vi "Data entry form multi-module.vi"(8 "error in (no error)":errorcluster, 9 "Assembly Type":string, 10 "Is Module?":bool, 11 "Database Entry in":refnum<class "Database Entry.lvclass">) -> (0 "error out":errorcluster, 1 "Is Dummy run?":bool, 2 "Aborted":bool, 3 "Database Entry out":refnum<class "Database Entry.lvclass">)   [LabVIEW 2021, in "Database Entry.lvclass"]
uses:
  Database Entry.lvclass
  Database Entry.lvclass/Database Entry.ctl
  Components/Stack/Stack.lvclass
panel:
  out "RingText.Text":string
  out "Now assembling...":string
  in  "Protomodule Steps":T1(ring)
  in  "Module Steps":T2(ring)
  in  "Dummy run submit":bool
  out "Use same values for both":bool
  in  "Use same values for all":bool
  out "Instructions":string
  in  "Module Instuctions":T3(ring)
  in  "Protomodule Instructions":T4(ring)
  in  "Submit":bool
  in  "Gantry":T5
  out "Stage":string
  in  "Steps":T6(ring)
  in  "Abort":bool
  in  "Next":bool
  in  "Previous":bool
  # "Col 1"
  # "Col 2"
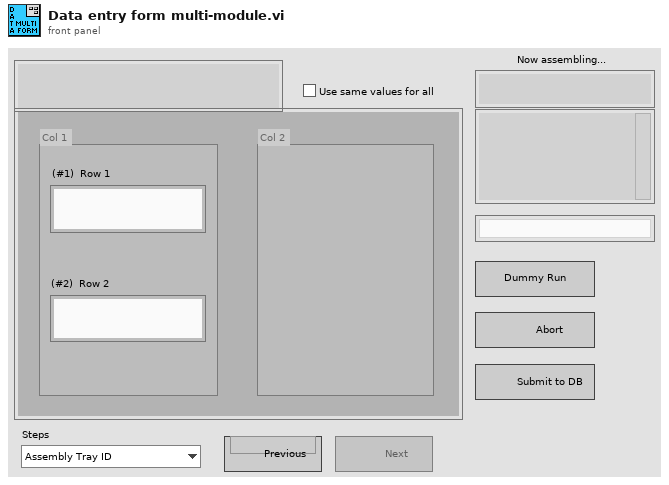
[diagram p1: front panel]
types:
  T1 = enum16{"Assembly Tray ID", "Module Stack ID", "Baseplate ID", "Sensor PUT ID", "Sensor Tray ID", "Sensor ID", "Sensor grade", "Comments", "Glue batch number", "Tape batch number"}
  T2 = enum16{"Assembly Tray ID", "Module Stack ID", "Protomodule ID", "Hexaboard PUT ID", "Hexaboard Tray ID", "Hexaboard ID", "Sensor grade", "Comments", "Glue batch number", "Tape batch number"}
  T3 = enum16{"Assembly Tray ID is always required.                For dummy runs, skip entry of other data.", "Scan the MODULE QR code (320M).                 **Leave blank for dummy runs**", "Verify the protomodule ID (320P) or scan the module QR code.                 **Leave blank for dummy runs**", "Hexaboard pick-up-tool ID", "Hexaboard Tray ID", "Scan the hexaboard QR code (320XL).                 **Leave blank for dummy runs**", "(Optional) Leave blank if no updated grade for the sensor", "Comments, if any.", "Glue batch number", "Tape batch number"}
  T4 = enum16{"Assembly Tray ID is always required.                For dummy runs, skip entry of other data.", "Scan the MODULE QR code (320M) for this protomodule.                 **Leave blank for dummy runs**", "Scan the baseplate QR code (320BA).                 **Leave blank for dummy runs**", "Sensor pick-up-tool ID", "Sensor Tray ID", "Scan the sensor barcode.                 **Leave blank for dummy runs**", "Sensor grade (default A)", "Include sensor visual inspection comments here.", "Glue batch number", "(Optional) Tape batch number"}
  T5 = cluster{"(#1)  Row 1":string, "(#2)  Row 2":string, "(#3)  Row 1":string, "(#4)  Row 2":string}
  T6 = enum16{"Assembly Tray ID", "Module Stack ID", "Base-layer (BP/PL) ID", "Pick-up-tool ID", "Component Tray ID", "Top-layer (Sen/Hxb) ID", "Sensor grade", "Comments", "Glue batch number"}
  T7 = enum8{"Enabled", "Disabled", "Disabled and Grayed Out"}
  T8 = enum16{"Assembly Tray ID", "Module Stack ID", "Base-layer (BP/PL) ID", "Pick-up-tool ID", "Component Tray ID", "Top-layer (Sen/Hxb) ID", "Sensor grade", "Comments", "Glue batch number", "Tape batch number"}
  T9 = cluster{"(#1)  Pos 1":string, "(#2)  Pos 2":string, "(#3)  Pos 1":string, "(#4)  Pos 2":string}
  T10 = cluster{"Value[0]":string, "Value[1]":string, "Value[2]":string, "Value[3]":string}
  T11 = cluster{"[0]":string, "[1]":string, "[2]":string, "[3]":string}
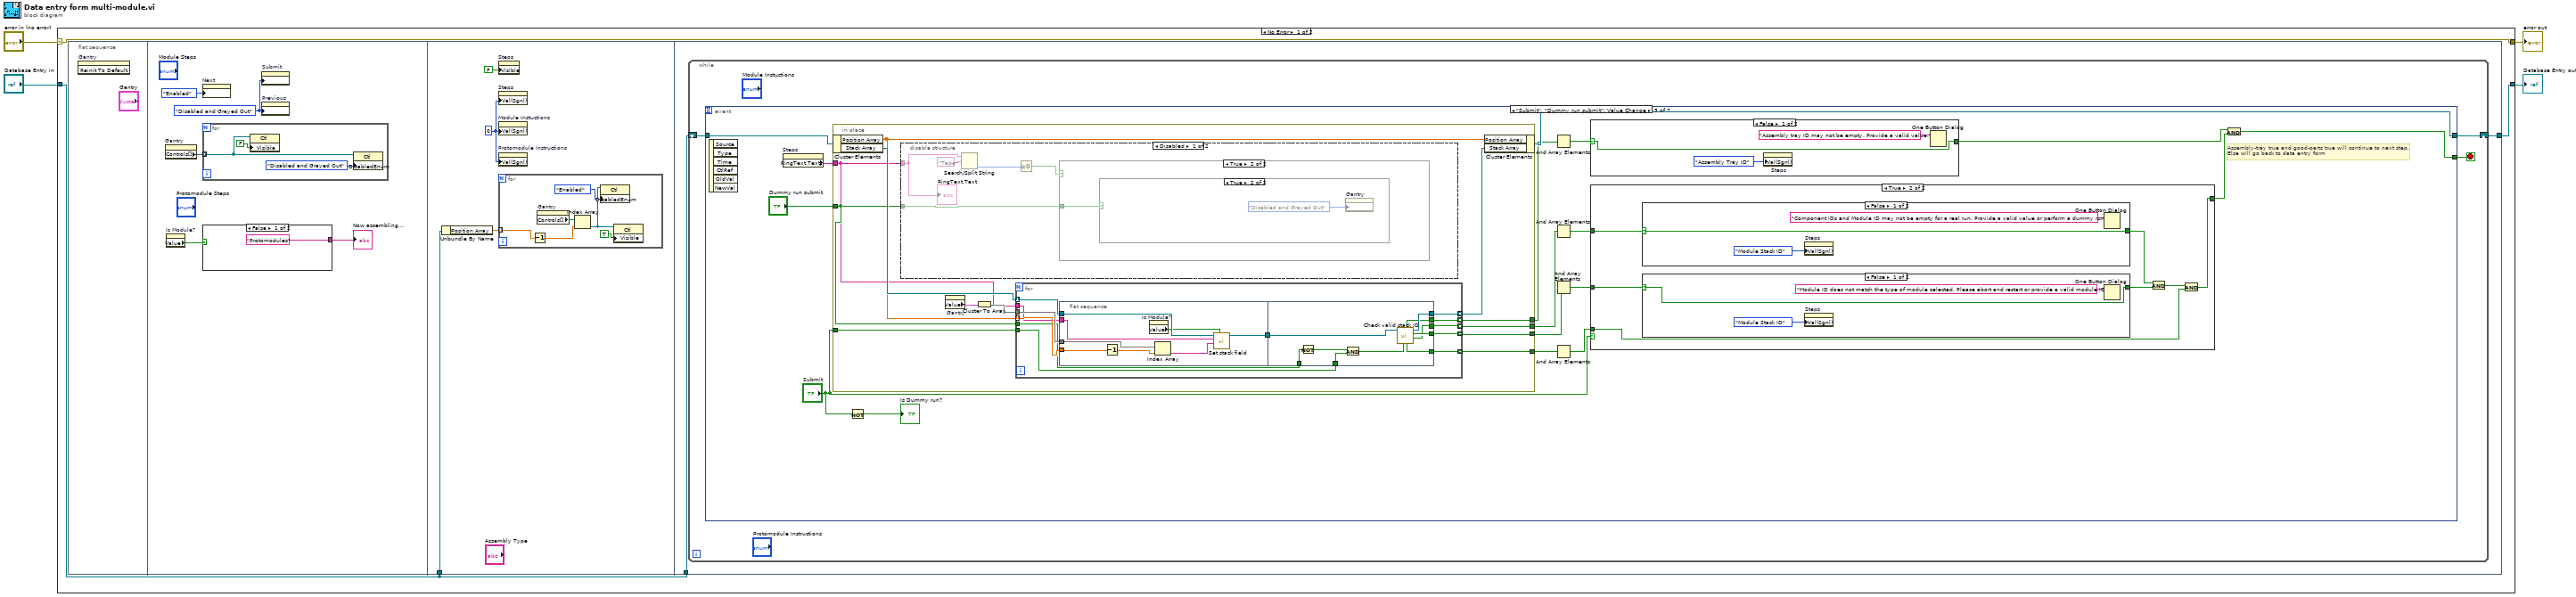
[diagram p0: block diagram]
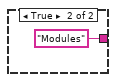
[diagram p2: hidden frame]
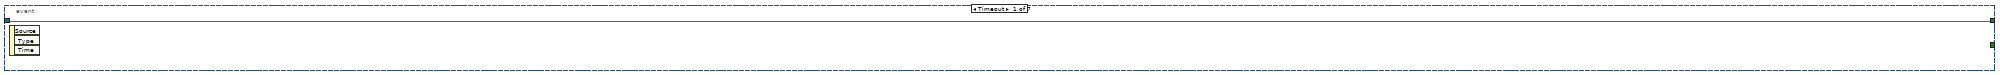
[diagram p3: hidden frame]
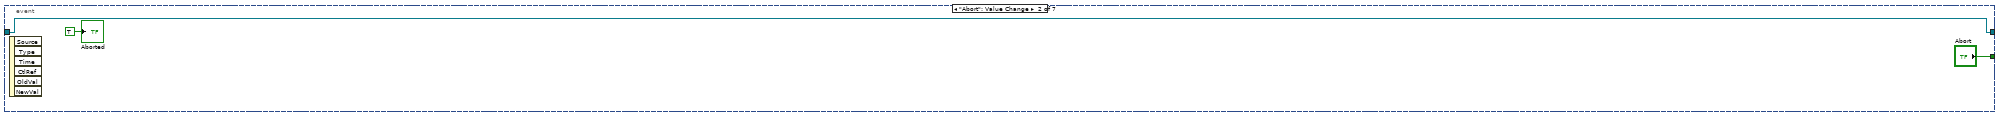
[diagram p4: hidden frame]
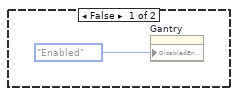
[diagram p5: hidden frame]
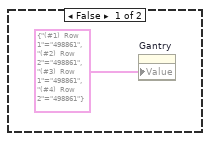
[diagram p6: hidden frame]
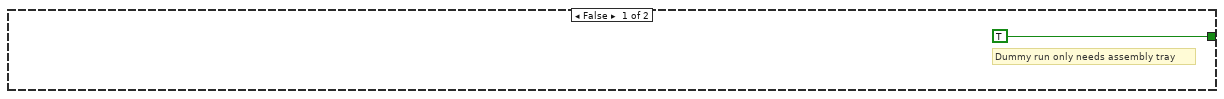
[diagram p8: hidden frame]
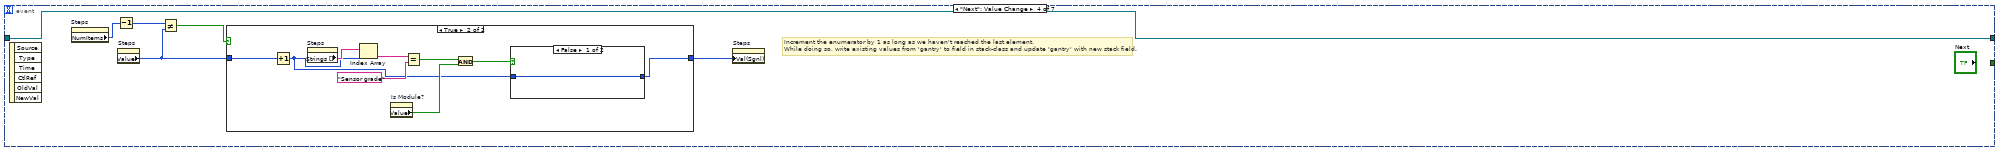
[diagram p12: hidden frame]
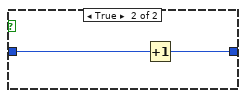
[diagram p14: hidden frame]
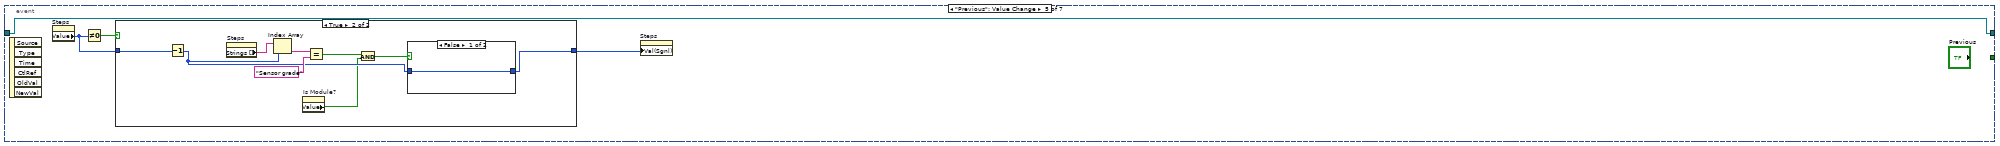
[diagram p15: hidden frame]
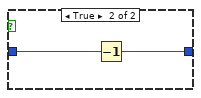
[diagram p17: hidden frame]
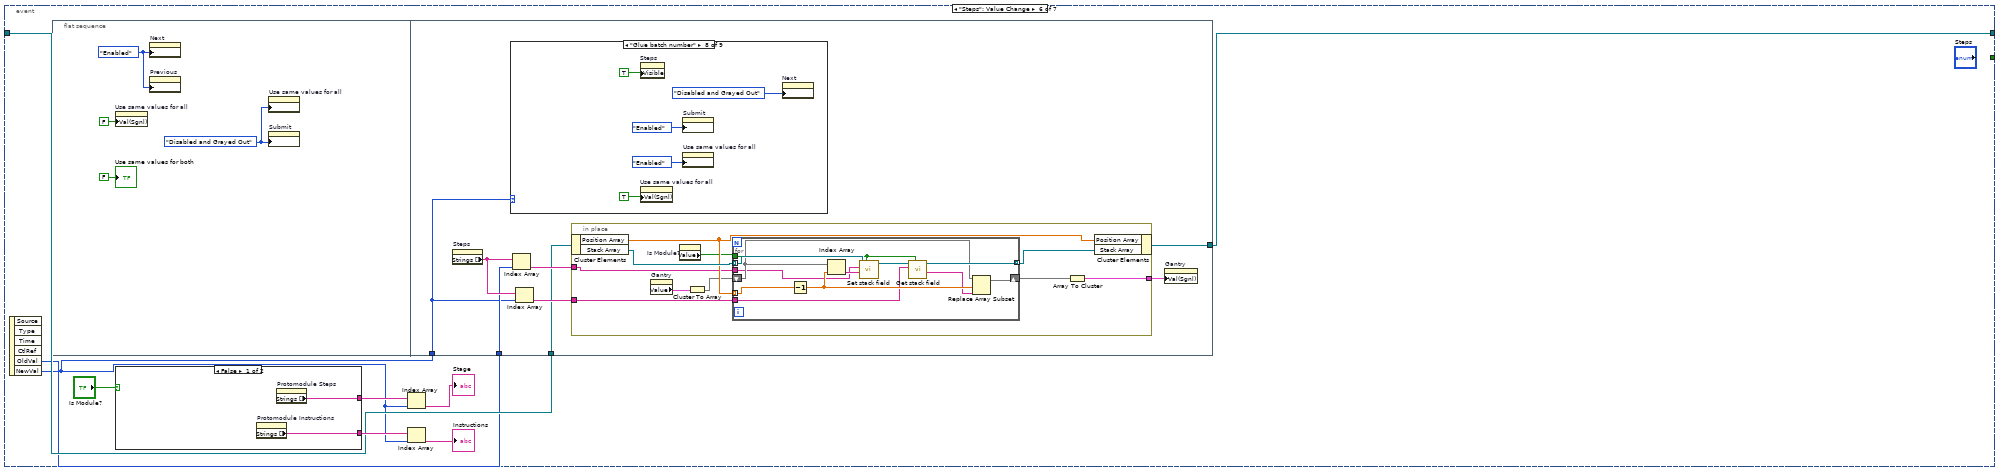
[diagram p18: hidden frame]
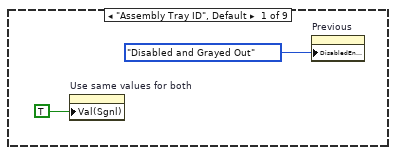
[diagram p19: hidden frame]
diagram:
  n1 = case shown="No Error" "error in (no error)" {
    selector: "error in (no error)" -> [w7 w298]
    tunnel: [w7 w298] -> w3
    tunnel: "Database Entry in" -> [w5 w297]
    tunnel: [w6 w297] -> w1
    frame No Error {
      n2 = flat-sequence {
        tunnel: w5 -> [w19]
        tunnel: w5 -> [w28]
        tunnel: [w29] -> w6
        frame #0 {
          n3 = invoke on="Gantry" class="Clust (strict)" method="Reinit To Default"() -> ()  [unwired: 3 in, 3 out]
        }
        frame #1 {
          w11 = T7."Disabled and Grayed Out" ("Disabled")
          n4 = property on="Gantry" class="Clust (strict)"() -> ("Controls[]"=w12:refnum<vi>[])  [unwired: 2 in, 2 out]
          n5 = property on="Is Module?" class="Bool (strict)"() -> ("Value"=w8:bool)  [unwired: 2 in, 2 out]
          n6 = property on="Next" class="Bool"("DisabledEnum"=T7."Enabled" ("Disabled")) -> ()  [unwired: 2 in, 2 out]
          n7 = for {
            tunnel: w12 -> [w15] mode=indexing
            n8 = property class="Ctl"(reference=w15, "Visible"=FALSE) -> ()  [unwired: 1 in, 2 out]
            n9 = property class="Ctl"(reference=w15, "DisabledEnum"=T7."Disabled and Grayed Out" ("Disabled")) -> ()  [unwired: 1 in, 2 out]
          }
          n10 = case shown="False" w8 {
            tunnel: ["Protomodules" ("Now assembling...") "Modules" ("Now assembling...")] -> w9
            frame False {
            }
            frame True {
            }
          }
          "Now assembling..." <- w9
          n11 = property on="Submit" class="Bool"("DisabledEnum"=w11) -> ()  [unwired: 2 in, 2 out]
          n12 = property on="Previous" class="Bool"("DisabledEnum"=w11) -> ()  [unwired: 2 in, 2 out]
        }
        frame #2 {
          w20 = u16 0 ("Value (Signaling)")
          n13 = Unbundle By Name(w19) -> ("Position Array"=w18:dbl[])
          n14 = property on="Steps" class="Enum (strict)"("Visible"=FALSE) -> ()  [unwired: 2 in, 2 out]
          n15 = property on="Steps" class="Enum (strict)"("Val(Sgnl)"=w20) -> ()  [unwired: 2 in, 2 out]
          n16 = property on="Module Instuctions" class="Enum (strict)"("Val(Sgnl)"=w20) -> ()  [unwired: 2 in, 2 out]
          n17 = property on="Protomodule Instructions" class="Enum (strict)"("Val(Sgnl)"=w20) -> ()  [unwired: 2 in, 2 out]
          n18 = for {
            tunnel: w18 -> [w23] mode=indexing
            n19 = Decrement(x=w23) -> (x-1=w22:dbl)
            n20 = property on="Gantry" class="Clust (strict)"() -> ("Controls[]"=w27:refnum<vi>[])  [unwired: 2 in, 2 out]
            n21 = Index Array(array=w27, index=w22) -> (element=w25:refnum<vi>)
            n22 = property class="Ctl"(reference=w25, "DisabledEnum"=T7."Enabled" ("Disabled")) -> ()  [unwired: 1 in, 2 out]
            n23 = property class="Ctl"(reference=w25, "Visible"=TRUE) -> ()  [unwired: 1 in, 2 out]
          }
        }
        frame #3 {
          n24 = while {
            shift-right: [w31] -> w29
            shift-left: w28 -> [w30]
            stop <- w32 stop-if-true
            # "While loop"
            n25 = event shown="[2] \"Submit\", \"Dummy run submit\": Value Change" {
              selector: _ -> [_ _ _ _ _ _ _]
              dyn-events: _ -> [_ _ _ _ _ _ _]
              timeout: _ -> [_ _ _ _ _ _ _]
              tunnel: [_ "Abort" w42 _ _ _ _] -> w32
              tunnel: w30 -> [w33 w35 w53 w125 w144 w164 w216]
              tunnel: [w33 w35 w52 w125 w144 w163 w216] -> w31
              event Timeout {
                n26 = event-data() -> ()  [unwired: 1 in, 3 out]
              }
              event "Abort": Value Change {
                n27 = event-data() -> ()  [unwired: 1 in, 6 out]
                "Aborted" <- TRUE ("Aborted")
              }
              event "Submit", "Dummy run submit": Value Change {
                # "Assembly-tray true and good-parts true will continue to next step. \nElse will go back to data entry form"
                n28 = event-data() -> ()  [unwired: 1 in, 6 out]
                n29 = property on="Steps" class="Enum (strict)"() -> ("RingText.Text"=w48:string)  [unwired: 2 in, 2 out]
                n30 = in-place {
                  in-place-border: w48 -> [w54]
                  in-place-border: [w60] -> w51
                  in-place-border: [w59] -> w50
                  in-place-border: [w58] -> w49
                  in-place-border: "Dummy run submit" -> [w57]
                  in-place-border: "Submit" -> [w56]
                  in-place-border: [w55] -> w38
                  n31 = in-place-cluster #1(w53) -> ("Position Array"=w64:dbl[], "Stack Array"=w65:refnum<class "Stack.lvclass">[])
                  n32 = disable-structure shown="Disabled" {
                    disable-tunnel: w57 -> [w70 _]
                    disable-tunnel: w54 -> [w69 _]
                    frame Disabled {
                      n33 = Search/Split String(string=w69, search string/char (-)="Tape") -> (offset of match=w67:i32)  [unwired: 1 in, 2 out]
                      n34 = Greater Or Equal To 0?(x=w67) -> (x >= 0?=w66:bool)
                      n35 = case shown="True" w66 {
                        tunnel: w70 -> [_ w72]
                        frame False {
                          n36 = property on="Gantry" class="Clust (strict)"("DisabledEnum"=T7."Enabled" ("Disabled")) -> ()  [unwired: 2 in, 2 out]
                        }
                        frame True {
                          n37 = case shown="True" w72 {
                            frame False {
                              n38 = property on="Gantry" class="Clust (strict)"("Value"=T5 {"(#1)  Row 1"="498861", "(#2)  Row 2"="498861", "(#3)  Row 1"="498861", "(#4)  Row 2"="498861"} ("Gantry")) -> ()  [unwired: 2 in, 2 out]
                            }
                            frame True {
                              n39 = property on="Gantry" class="Clust (strict)"("DisabledEnum"=T7."Disabled and Grayed Out" ("Disabled")) -> ()  [unwired: 2 in, 2 out]
                            }
                          }
                        }
                      }
                      "RingText.Text" <- w69
                    }
                    frame Enabled {
                    }
                  }
                  n40 = property on="Gantry" class="Clust (strict)"() -> ("Value"=w62:T9)  [unwired: 2 in, 2 out]
                  n41 = Cluster To Array(cluster=w62) -> (array=w63:string[])
                  n42 = for {
                    tunnel: w65 -> [w86] mode=indexing
                    tunnel: w64 -> [w85] mode=indexing
                    tunnel: [w83] -> w61 mode=indexing
                    tunnel: w54 -> [w76]
                    tunnel: w63 -> [w84]
                    tunnel: w56 -> [w81]
                    tunnel: w57 -> [w75]
                    tunnel: [w80] -> w60 mode=indexing
                    tunnel: [w79] -> w59 mode=indexing
                    tunnel: [w78] -> w58 mode=indexing
                    tunnel: [w77] -> w55 mode=indexing
                    n43 = flat-sequence {
                      tunnel: w86 -> [w94]
                      tunnel: w85 -> [w93]
                      tunnel: w84 -> [w91]
                      tunnel: w76 -> [w89]
                      tunnel: [w88] -> w82
                      tunnel: [w103] -> w83
                      tunnel: w82 -> [w104]
                      tunnel: w81 -> [w101]
                      tunnel: w75 -> [w100]
                      tunnel: [w98] -> w80
                      tunnel: [w97] -> w79
                      tunnel: [w96] -> w78
                      tunnel: [w95] -> w77
                      frame #0 {
                        n44 = Decrement(x=w93) -> (x-1=w90:dbl)
                        n45 = property on="Is Module?" class="Bool (strict)"() -> ("Value"=w87:bool)  [unwired: 2 in, 2 out]
                        n46 = Index Array(array=w91, index=w90) -> (element=w92:string)
                        n47 = call "Set stack field.vi"("Is Module?"=w87, "Value in"=w92, "Field"=w89, "Stack in"=w94) -> ("Stack out"=w88:refnum<class "Stack.lvclass">)  [unwired: 6 in, 1 out]
                      }
                      frame #1 {
                        n48 = Not(x=w100) -> (.not. x?=w99:bool)
                        n49 = And(x=w99, y=w101) -> (x .and. y?=w102:bool)
                        n50 = call "Check valid stack ID.vi"("Is real run?"=w102, "Stack in"=w104) -> ("Non-empty part IDs?"=w97:bool, "Valid module ID?"=w98:bool, "Stack out"=w103:refnum<class "Stack.lvclass">, "Continue with current parts"=w95:bool, "Non-empty assembly tray ID?"=w96:bool)  [unwired: 4 in, 1 out]
                      }
                    }
                  }
                  n51 = in-place-cluster #1("Position Array"=w64, "Stack Array"=w61) -> (w52:refnum<class "Database Entry.lvclass">)
                }
                n52 = Not(x="Submit") -> (.not. x?=→"Is Dummy run?":bool)
                n53 = And Array Elements(Boolean array=w49) -> (logical AND=w47:bool)
                n54 = And Array Elements(Boolean array=w50) -> (logical AND=w46:bool)
                n55 = And Array Elements(Boolean array=w51) -> (logical AND=w44:bool)
                n56 = And Array Elements(Boolean array=w38) -> (logical AND=w37:bool)
                n57 = case shown="False" w47 {
                  selector: w47 -> [w122 w124]
                  tunnel: [w122 w124] -> w43
                  frame False {
                    n58 = property on="Steps" class="Enum (strict)"("Val(Sgnl)"=T8."Assembly Tray ID" ("Value (Signaling)")) -> ()  [unwired: 2 in, 2 out]
                    n59 = One Button Dialog(message="Assembly tray ID may not be empty. Provide a valid value.") -> ()  [unwired: 1 in, 1 out]
                  }
                  frame True {
                  }
                }
                n60 = case shown="True" "Submit" {
                  tunnel: w46 -> [_ w112]
                  tunnel: w44 -> [_ w111]
                  tunnel: [TRUE w106] -> w41
                  tunnel: w37 -> [_ w108]
                  frame False {
                    # "Dummy run only needs assembly tray"
                  }
                  frame True {
                    n61 = case shown="False" w112 {
                      selector: w112 -> [w118 w120]
                      tunnel: [w118 w120] -> w110
                      frame False {
                        n62 = property on="Steps" class="Enum (strict)"("Val(Sgnl)"=T8."Module Stack ID" ("Value (Signaling)")) -> ()  [unwired: 2 in, 2 out]
                        n63 = One Button Dialog(message="Component IDs and Module ID may not be empty for a real run. Provide a valid value or perform a dummy run.") -> ()  [unwired: 1 in, 1 out]
                      }
                      frame True {
                      }
                    }
                    n64 = case shown="False" w111 {
                      selector: w111 -> [w114 w116]
                      tunnel: [w114 w116] -> w109
                      frame False {
                        n65 = property on="Steps" class="Enum (strict)"("Val(Sgnl)"=T8."Module Stack ID" ("Value (Signaling)")) -> ()  [unwired: 2 in, 2 out]
                        n66 = One Button Dialog(message="Module ID does not match the type of module selected. Please abort and restart or provide a valid module ID.") -> ()  [unwired: 1 in, 1 out]
                      }
                      frame True {
                      }
                    }
                    n67 = And(x=w110, y=w109) -> (x .and. y?=w107:bool)
                    n68 = And(x=w107, y=w108) -> (x .and. y?=w106:bool)
                  }
                }
                n69 = And(x=w43, y=w41) -> (x .and. y?=w42:bool)
              }
              event "Next": Value Change {
                # "Increment the enumerator by 1 as long as we haven't reached the last element.\nWhile doing so, write existing values from 'gantry' to field in stack-class and update 'gantry' with new stack field."
                n70 = event-data() -> ()  [unwired: 1 in, 6 out]
                n71 = property on="Steps" class="Enum (strict)"() -> ("NumItems"=w130:u32)  [unwired: 2 in, 2 out]
                n72 = Decrement(x=w130) -> (x-1=w129:u32)
                n73 = property on="Steps" class="Enum (strict)"() -> ("Value"=w127:T6)  [unwired: 2 in, 2 out]
                n74 = Not Equal?(x=w129, y=w127) -> (x != y?=w128:bool)
                n75 = case shown="True" w128 {
                  tunnel: w127 -> [w131 w140]
                  tunnel: [w131 w132] -> w126
                  frame False {
                  }
                  frame True {
                    n76 = Increment(x=w140) -> (x+1=w133:T6)
                    n77 = property on="Steps" class="Enum (strict)"() -> ("Strings []"=w139:string[])  [unwired: 2 in, 2 out]
                    n78 = Index Array(array=w139, index=w133) -> (element=w138:string)
                    n79 = property on="Is Module?" class="Bool (strict)"() -> ("Value"=w135:bool)  [unwired: 2 in, 2 out]
                    n80 = Equal?(x=w138, y="Sensor grade") -> (x = y?=w136:bool)
                    n81 = And(x=w136, y=w135) -> (x .and. y?=w134:bool)
                    n82 = case shown="False" w134 {
                      tunnel: w133 -> [w141 w143]
                      tunnel: [w141 w142] -> w132
                      frame False {
                      }
                      frame True {
                        n83 = Increment(x=w143) -> (x+1=w142:T6)
                      }
                    }
                  }
                }
                n84 = property on="Steps" class="Enum (strict)"("Val(Sgnl)"=w126) -> ()  [unwired: 2 in, 2 out]
              }
              event "Previous": Value Change {
                n85 = event-data() -> ()  [unwired: 1 in, 6 out]
                n86 = property on="Steps" class="Enum (strict)"() -> ("Value"=w146:T6)  [unwired: 2 in, 2 out]
                n87 = Not Equal To 0?(x=w146) -> (x != 0?=w147:bool)
                n88 = case shown="True" w147 {
                  tunnel: w146 -> [w148 w157]
                  tunnel: [w148 w149] -> w145
                  frame False {
                  }
                  frame True {
                    n89 = Decrement(x=w157) -> (x-1=w152:T6)
                    n90 = property on="Steps" class="Enum (strict)"() -> ("Strings []"=w151:string[])  [unwired: 2 in, 2 out]
                    n91 = Index Array(array=w151, index=w152) -> (element=w156:string)
                    n92 = property on="Is Module?" class="Bool (strict)"() -> ("Value"=w150:bool)  [unwired: 2 in, 2 out]
                    n93 = Equal?(x=w156, y="Sensor grade") -> (x = y?=w154:bool)
                    n94 = And(x=w154, y=w150) -> (x .and. y?=w153:bool)
                    n95 = case shown="False" w153 {
                      tunnel: w152 -> [w158 w160]
                      tunnel: [w158 w159] -> w149
                      frame False {
                      }
                      frame True {
                        n96 = Decrement(x=w160) -> (x-1=w159:T6)
                      }
                    }
                  }
                }
                n97 = property on="Steps" class="Enum (strict)"("Val(Sgnl)"=w145) -> ()  [unwired: 2 in, 2 out]
              }
              event "Steps": Value Change {
                n98 = event-data() -> ("OldVal"=w162:T6, "NewVal"=w161:T6)  [unwired: 1 in, 4 out]
                n99 = flat-sequence {
                  tunnel: [w176] -> w163
                  tunnel: w164 -> [w177]
                  tunnel: w162 -> [w175]
                  tunnel: w161 -> [w174]
                  frame #0 {
                    w173 = T7."Disabled and Grayed Out" ("Disabled")
                    w172 = T7."Enabled" ("Disabled")
                    n100 = property on="Use same values for all" class="Bool (strict)"("Val(Sgnl)"=FALSE ("Value (Signaling)")) -> ()  [unwired: 2 in, 2 out]
                    n101 = property on="Next" class="Bool"("DisabledEnum"=w172) -> ()  [unwired: 2 in, 2 out]
                    n102 = property on="Previous" class="Bool"("DisabledEnum"=w172) -> ()  [unwired: 2 in, 2 out]
                    n103 = property on="Use same values for all" class="Bool (strict)"("DisabledEnum"=w173) -> ()  [unwired: 2 in, 2 out]
                    n104 = property on="Submit" class="Bool"("DisabledEnum"=w173) -> ()  [unwired: 2 in, 2 out]
                    "Use same values for both" <- FALSE ("Use same values for both")
                  }
                  frame #1 {
                    n105 = property on="Steps" class="Enum (strict)"() -> ("Strings []"=w178:string[])  [unwired: 2 in, 2 out]
                    n106 = case shown="\"Glue batch number\"" w174 {
                      frame "Assembly Tray ID", Default {
                        n107 = property on="Use same values for both" class="Bool (strict)"("Val(Sgnl)"=TRUE ("Value (Signaling)")) -> ()  [unwired: 2 in, 2 out]
                        n108 = property on="Previous" class="Bool"("DisabledEnum"=T7."Disabled and Grayed Out" ("Disabled")) -> ()  [unwired: 2 in, 2 out]
                      }
                      frame "Module Stack ID" {
                      }
                      frame "Base-layer (BP/PL) ID" {
                      }
                      frame "Pick-up-tool ID" {
                      }
                      frame "Component Tray ID" {
                        n109 = property on="Use same values for both" class="Bool (strict)"("Val(Sgnl)"=TRUE ("Value (Signaling)")) -> ()  [unwired: 2 in, 2 out]
                      }
                      frame "Top-layer (Sen/Hxb) ID" {
                      }
                      frame "Comments" {
                      }
                      frame "Glue batch number" {
                        n110 = property on="Steps" class="Enum (strict)"("Visible"=TRUE) -> ()  [unwired: 2 in, 2 out]
                        n111 = property on="Use same values for all" class="Bool (strict)"("Val(Sgnl)"=TRUE ("Value (Signaling)")) -> ()  [unwired: 2 in, 2 out]
                        n112 = property on="Submit" class="Bool"("DisabledEnum"=T7."Enabled" ("Disabled")) -> ()  [unwired: 2 in, 2 out]
                        n113 = property on="Use same values for all" class="Bool (strict)"("DisabledEnum"=T7."Enabled" ("Disabled")) -> ()  [unwired: 2 in, 2 out]
                        n114 = property on="Next" class="Bool"("DisabledEnum"=T7."Disabled and Grayed Out" ("Disabled")) -> ()  [unwired: 2 in, 2 out]
                      }
                      frame "Sensor grade" {
                      }
                    }
                    n115 = Index Array(array=w178, index=w175) -> (element=w179:string)
                    n116 = Index Array(array=w178, index=w174) -> (element=w180:string)
                    n117 = in-place {
                      in-place-border: w179 -> [w195]
                      in-place-border: w180 -> [w194]
                      in-place-border: [w190] -> w181
                      n118 = in-place-cluster #2(w177) -> ("Position Array"=w198:dbl[], "Stack Array"=w199:refnum<class "Stack.lvclass">[])
                      n119 = property on="Gantry" class="Clust (strict)"() -> ("Value"=w193:T9)  [unwired: 2 in, 2 out]
                      n120 = property on="Is Module?" class="Bool (strict)"() -> ("Value"=w192:bool)  [unwired: 2 in, 2 out]
                      n121 = Cluster To Array(cluster=w193) -> (array=w196:string[])
                      n122 = for {
                        tunnel: w199 -> [w211] mode=indexing
                        tunnel: w198 -> [w210] mode=indexing
                        tunnel: [w209] -> w197 mode=indexing
                        tunnel: w195 -> [w202]
                        tunnel: w194 -> [w201]
                        tunnel: w192 -> [w200]
                        shift-right: [w203] -> w191
                        shift-left: w196 -> [w206]
                        n123 = Decrement(x=w210) -> (x-1=w205:dbl)
                        n124 = Index Array(array=w206, index=w205) -> (element=w207:string)
                        n125 = call "Set stack field.vi"("Is Module?"=w200, "Value in"=w207, "Field"=w202, "Stack in"=w211) -> ("Stack out"=w208:refnum<class "Stack.lvclass">)  [unwired: 6 in, 1 out]
                        n126 = call "Get stack field.vi"("Is Module?"=w200, "Field"=w201, "Stack in"=w208) -> ("Value out"=w204:string, "Stack out"=w209:refnum<class "Stack.lvclass">)  [unwired: 6 in, 1 out]
                        n127 = Replace Array Subset(array=w206, new element=w204, index=w205) -> (w203:string[])
                      }
                      n128 = Array To Cluster(array=w191) -> (cluster=w190:T10)
                      n129 = in-place-cluster #2("Position Array"=w198, "Stack Array"=w197) -> (w176:refnum<class "Database Entry.lvclass">)
                    }
                    n130 = property on="Gantry" class="Clust (strict)"("Val(Sgnl)"=w181) -> ()  [unwired: 2 in, 2 out]
                  }
                }
                n131 = case shown="False" "Is Module?" {
                  tunnel: [w213 w215] -> w169
                  tunnel: [w212 w214] -> w165
                  frame False {
                    n132 = property on="Protomodule Instructions" class="Enum (strict)"() -> ("Strings []"=w213:string[])  [unwired: 2 in, 2 out]
                    n133 = property on="Protomodule Steps" class="Enum (strict)"() -> ("Strings []"=w212:string[])  [unwired: 2 in, 2 out]
                  }
                  frame True {
                    n134 = property on="Module Instuctions" class="Enum (strict)"() -> ("Strings []"=w215:string[])  [unwired: 2 in, 2 out]
                    n135 = property on="Module Steps" class="Enum (strict)"() -> ("Strings []"=w214:string[])  [unwired: 2 in, 2 out]
                  }
                }
                n136 = Index Array(array=w165, index=w161) -> (element=→"Stage":string)
                n137 = Index Array(array=w169, index=w161) -> (element=→"Instructions":string)
              }
              event "Gantry": Value Change {
                n138 = event-data() -> ("OldVal"=w219:T5, "NewVal"=w218:T5)  [unwired: 1 in, 4 out]
                n139 = property on="Use same values for both" class="Bool (strict)"() -> ("Value"=w217:bool)  [unwired: 2 in, 2 out]
                n140 = case shown="False" "Use same values for all" {
                  tunnel: w218 -> [_ w281]
                  tunnel: w219 -> [_ w279]
                  frame False {
                  }
                  frame True {
                    # "If all strings have same value, do nothing. If false, make them same."
                    n141 = Cluster To Array(cluster=w279) -> (array=w280:string[])
                    n142 = Cluster To Array(cluster=w281) -> (array=w278:string[])
                    n143 = Index Array(array=w278) -> (element=w277:string)  [unwired: 1 in]
                    n144 = Equal?(x=w278, y=w277) -> (x = y?=w276:bool[])
                    n145 = And Array Elements(Boolean array=w276) -> (logical AND=w275:bool)
                    n146 = case shown="False" w275 {
                      tunnel: w280 -> [w288 _]
                      tunnel: w278 -> [w285 _]
                      frame False {
                        n147 = Not Equal?(x=w288, y=w285) -> (x != y?=w291:bool[])
                        n148 = Array Size(array=w285) -> (size(s)=w287:i32)
                        n149 = Search 1D Array(1D array=w291, element=TRUE) -> (index of element=w290:i32)  [unwired: 1 in]
                        n150 = Index Array(array=w285, index=w290) -> (element=w289:string)
                        n151 = for {
                          N: w287 -> [_]
                          tunnel: w289 -> [w294]
                          shift-right: [w295] -> w284
                          shift-left: string[] [] -> [w293]
                          i -> [w296]
                          n152 = Insert Into Array(array=w293, index=w296, new element=w294) -> (w295:string[])
                        }
                        n153 = Array Subset(array=w284, length=w287) -> (w283:string[])  [unwired: 1 in]
                        n154 = Array To Cluster(array=w283) -> (cluster=w286:T11)
                        n155 = property on="Gantry" class="Clust (strict)"("Val(Sgnl)"=w286) -> ()  [unwired: 2 in, 2 out]
                      }
                      frame True {
                      }
                    }
                  }
                }
                n156 = case shown="True" w217 {
                  tunnel: w218 -> [_ w229]
                  tunnel: w219 -> [_ w228]
                  frame False {
                  }
                  frame True {
                    # "no of trays"
                    n157 = Cluster To Array(cluster=w228) -> (array=w223:string[])
                    n158 = Cluster To Array(cluster=w229) -> (array=w222:string[])
                    n159 = Array Size(array=w222) -> (size(s)=w227:i32)
                    n160 = Divide(x=w227, y=2) -> (x/y=w225:dbl)
                    n161 = for {
                      N: w225 -> [_]
                      tunnel: w222 -> [w234]
                      tunnel: [w233] -> w221 mode=indexing
                      i -> [w232]
                      # "The two positions in a given tray have same tray id value. If false, set them to have same value"
                      n162 = Multiply(x=2 ("y"), y=w232) -> (x*y=w230:i32)
                      n163 = Increment(x=w230) -> (x+1=w237:i32)
                      n164 = Index Array(array=w234, index #1=w230, index #2=w237) -> (element #1=w235:string, element #2=w236:string)
                      n165 = Equal?(x=w235, y=w236) -> (x = y?=w233:bool)
                    }
                    n166 = And Array Elements(Boolean array=w221) -> (logical AND=w224:bool)
                    n167 = case shown="True" w224 {
                      tunnel: w223 -> [w241 _]
                      tunnel: w222 -> [w245 _]
                      tunnel: w225 -> [w246 _]
                      tunnel: w221 -> [w238 _]
                      frame False {
                        n168 = Array Size(array=w241) -> (size(s)=w242:i32)
                        n169 = for {
                          N: w246 -> [_]
                          tunnel: w241 -> [w252]
                          tunnel: w245 -> [w250]
                          shift-right: [w248] -> w243
                          shift-left: string[] [] -> [w249]
                          tunnel: w238 -> [w247] mode=indexing
                          i -> [w251]
                          # "If the two positions in a tray have diff values, make them same. Else retain original values"
                          n170 = case shown="True" w247 {
                            tunnel: w252 -> [w265 _]
                            tunnel: w251 -> [w264 w271]
                            tunnel: w250 -> [w263 w272]
                            tunnel: w249 -> [w256 w270]
                            tunnel: [w255 w267] -> w248
                            frame False {
                              w262 = 2 ("length")
                              n171 = Multiply(x=2 ("y"), y=w264) -> (x*y=w254:i32)
                              n172 = Array Subset(array=w265, index=w254, length=w262) -> (w261:string[])
                              n173 = Array Subset(array=w263, index=w254, length=w262) -> (w258:string[])
                              n174 = Not Equal?(x=w261, y=w258) -> (x != y?=w260:bool[])
                              n175 = Search 1D Array(1D array=w260, element=TRUE) -> (index of element=w257:i32)  [unwired: 1 in]
                              n176 = Index Array(array=w258, index=w257) -> (element=w253:string)
                              n177 = Insert Into Array(array=w256, index=w254, new element #1=w253, new element #2=w253) -> (w255:string[])
                            }
                            frame True {
                              n178 = Multiply(x=2 ("y"), y=w271) -> (x*y=w269:i32)
                              n179 = Array Subset(array=w272, index=w269, length=2) -> (w268:string[])
                              n180 = Insert Into Array(array=w270, index=w269, new element=w268) -> (w267:string[])
                            }
                          }
                        }
                        n181 = Array Subset(array=w243, length=w242) -> (w240:string[])  [unwired: 1 in]
                        n182 = Array To Cluster(array=w240) -> (cluster=w239:T11)
                        n183 = property on="Gantry" class="Clust (strict)"("Val(Sgnl)"=w239) -> ()  [unwired: 2 in, 2 out]
                      }
                      frame True {
                      }
                    }
                  }
                }
              }
            }
          }
        }
      }
    }
    frame Error {
    }
  }
  "error out" <- w3
  "Database Entry out" <- w1
